vi "AppendWaveformRead.vi"(10 "WFM in":T1, 11 "index of element":i32) -> (3 "WFM out":T1)   [LabVIEW 2016]
uses:
  SMOs/DAQ/Typedefs/PublicEvents--DAQ.Read.ctl
  SMOs/DAQ/DAQ.lvclass
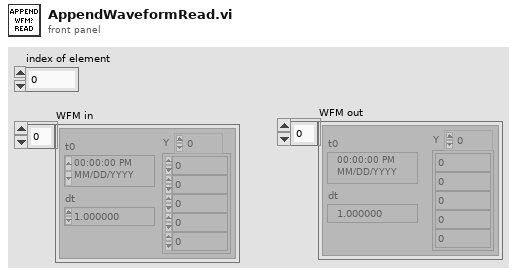
[diagram p1: front panel]
types:
  T1 = typedef "DAQ.lvclass/PublicEvents--DAQ.Read.ctl" = waveform(dbl)[]
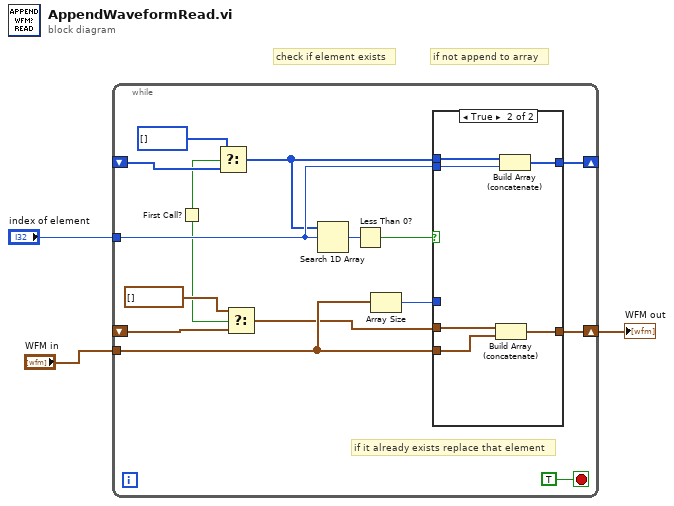
[diagram p0: block diagram]
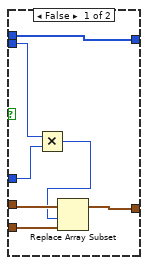
[diagram p2: hidden frame]
diagram:
  # "if not append to array"
  # "check if element exists"
  n1 = while {
    tunnel: "WFM in" -> [w12]
    tunnel: "index of element" -> [w16]
    shift-right: [w17] -> _
    shift-left: _ -> [w6]
    shift-right: [w14] -> w1
    shift-left: _ -> [w9]
    stop <- TRUE stop-if-true
    # "if it already exists replace that element"
    n2 = First Call?() -> (First Call?: T/F=w4:bool)
    n3 = Select(t=i32[] [], s=w4, f=w6) -> (s? t:f=w5:i32[])
    n4 = Select(t=T1 [], s=w4, f=w9) -> (s? t:f=w8:T1)
    n5 = Search 1D Array(1D array=w5, element=w16) -> (index of element=w15:i32)  [unwired: 1 in]
    n6 = Less Than 0?(x=w15) -> (x < 0?=w13:bool)
    n7 = Array Size(array=w12) -> (size(s)=w11:i32)
    n8 = case shown="True" w13 {
      tunnel: [w19 w31] -> w17
      tunnel: w16 -> [w22 w30]
      tunnel: w5 -> [w19 w29]
      tunnel: w12 -> [w24 w28]
      tunnel: [w23 w27] -> w14
      tunnel: w8 -> [w25 w26]
      tunnel: w11 -> [w21 _]
      frame False {
        n9 = Multiply(x=w22, y=w21) -> (x*y=w20:i32)
        n10 = Replace Array Subset(array=w25, new element=w24, index=w20) -> (w23:T1)
      }
      frame True {
        n11 = Build Array (concatenate)(w26, w28) -> (w27:T1)
        n12 = Build Array (concatenate)(w29, w30) -> (w31:i32[])
      }
    }
  }
  "WFM out" <- w1
